vi "niRFUtil FWK Get Driver Validation from Database.vi"(8 "error in (no error)":errorcluster, 10 "Loaded Driver Type":T1, 11 "Driver Validation Database In":variant) -> (0 "error out":errorcluster, 2 "Valid Driver?":bool, 3 "Driver Validation Database Out":variant)   [LabVIEW 2015, in "niRFUtil.lvlib"]
uses:
  niRFUtil.lvlib
  Includes/niRFUtil INC FWK Class Types.ctl
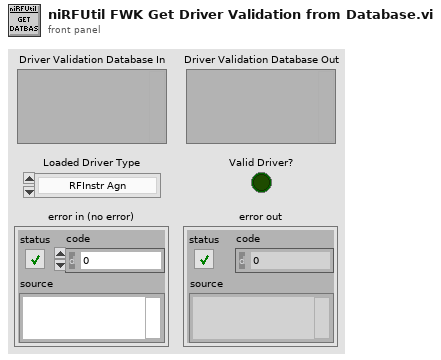
[diagram p1: front panel]
types:
  T1 = typedef "niRFUtil.lvlib/niRFUtil INC FWK Class Types.ctl" = enum16{"RFInstr Agn", "RFSAInstr", "DCPowerInstr"}
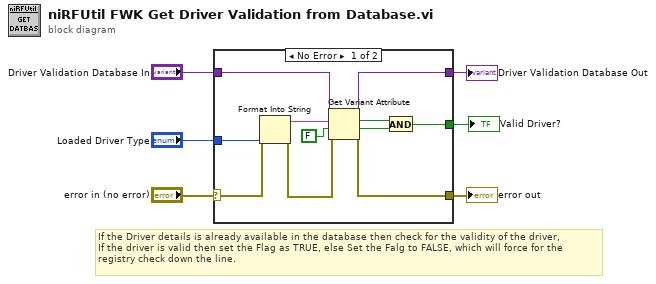
[diagram p0: block diagram]
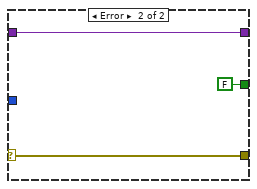
[diagram p2: hidden frame]
diagram:
  # "If the Driver details is already available in the database then check for the validity of the driver,\nIf the driver is valid then set the Flag as TRUE, else Set the Falg to FALSE, which will force for the \nregistry check down the line."
  n1 = case shown="No Error" "error in (no error)" {
    selector: "error in (no error)" -> [w8 w19]
    tunnel: "Driver Validation Database In" -> [w17 w20]
    tunnel: [w16 w20] -> w5
    tunnel: "Loaded Driver Type" -> [w15 _]
    tunnel: [w12 w19] -> w3
    tunnel: [w9 FALSE] -> w1
    frame No Error {
      n2 = Format Into String(error in=w8, w15) -> (resulting string=w14:string, error out=w7:errorcluster)  [unwired: 2 in]
      n3 = Get Variant Attribute(Variant=w17, name=w14, default value (empty Variant)=FALSE ("Valid Driver?"), error in=w7) -> (duplicate Variant=w16:variant, found=w11:bool, value=w10:bool, error out=w12:errorcluster)
      n4 = And(x=w11, y=w10) -> (x .and. y?=w9:bool)
    }
    frame Error {
    }
  }
  "error out" <- w3
  "Driver Validation Database Out" <- w5
  "Valid Driver?" <- w1
